vi "GL Center.vi"(5 "Simple":bool, 6 "error in":errorcluster, 8 "Axis":T1 items=["Axis 1", "Axis 2", "Axis 3", "Axis 4", "Axis 5", "Axis 6", "Axis 7", "Axis 8"], 9 "Galil.IGalil":refnum<k7>) -> (0 "error out":errorcluster, 2 "Axis Out":T1 items=["Axis 1", "Axis 2", "Axis 3", "Axis 4", "Axis 5", "Axis 6", "Axis 7", "Axis 8"], 3 "Galil Out":refnum<k7>)   [LabVIEW 2022 SP3]
doc: "Sets the operation mode for an axis or vector space."
uses:
  GL Axis Control.ctl
  Command Menu.ctl
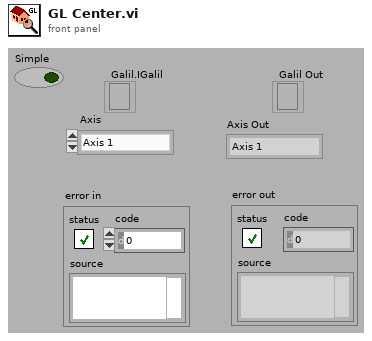
[diagram p1: front panel]
types:
  T1 = typedef "GL Axis Control.ctl" = u16
  T2 = enum16{"Absolute Position", "Relative Position", "Velocity", "Relative to Cap Pos", "Modulus Position", "Absolute Contouring", "Relative Contouring"}
  T3 = typedef "Command Menu.ctl" = enum16{"CommandPassThrough", "Abort Motion", "Define Pos", "Velocity", "Acceleration", "Deceleration", "Position Rel", "Postion Abs", "Begin Move", "After Move", "Home", "KI", "KD", "KP", "IL", "Config I/O", "Set Bit", "Clear Bit", "Motor Off", "Moto On", "Status", "Execute", "Halt Execute", "HX Status", "Tell Velocity", "Check Motion", "BreakPoint", "Tell Position", "Current Code Line", "Tell Switches", "OC Force On", "OC Off", "Pos Soft Limit", "Rev Soft Limit"}
  T4 = cluster{"HomeStatus":bool, "ReverseLimit?":bool, "ForwardLimit?":bool, "LimitHit?":bool, "MotorOff?":bool, "Motion?":bool}
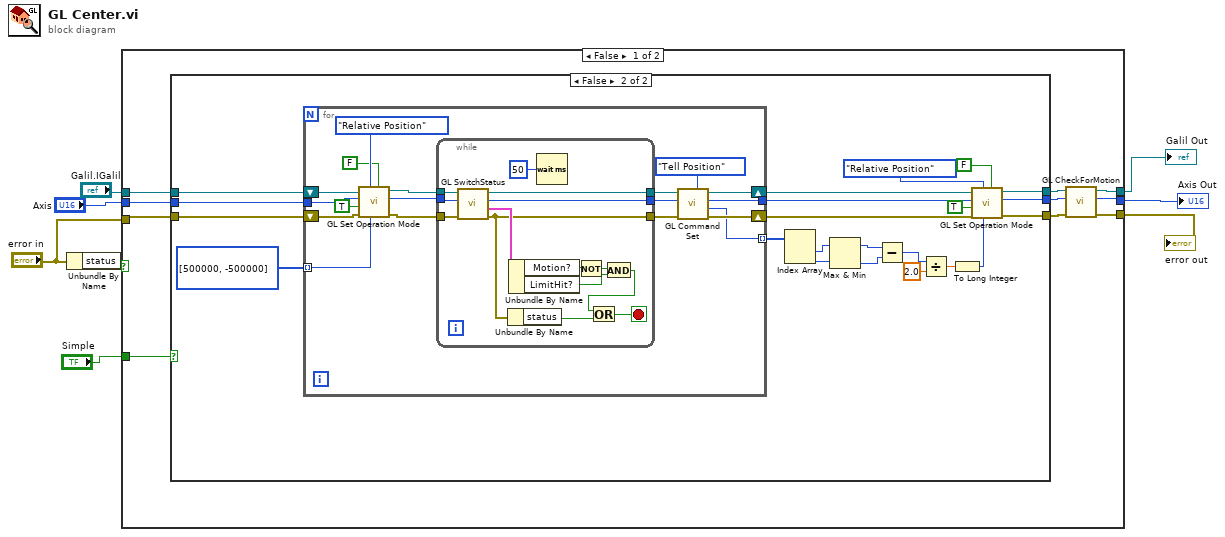
[diagram p0: block diagram]
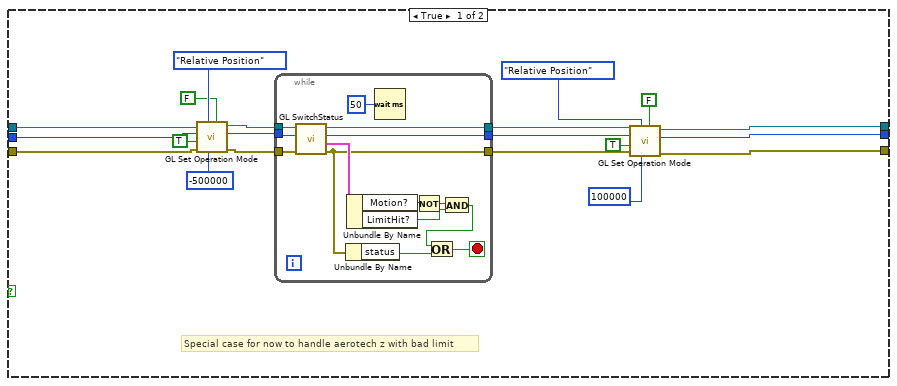
[diagram p2: hidden frame]
diagram:
  n1 = Unbundle By Name("error in") -> ("status"=w7:bool)
  n2 = case shown="False" w7 {
    tunnel: "error in" -> [w18 w109]
    tunnel: [w11 w109] -> w8
    tunnel: [w12 w108] -> w6
    tunnel: "Galil.IGalil" -> [w17 w108]
    tunnel: "Axis" -> [w16 w107]
    tunnel: [w10 w107] -> w3
    tunnel: "Simple" -> [w15 _]
    frame False {
      n3 = case shown="False" w15 {
        tunnel: w18 -> [w38 w74]
        tunnel: w17 -> [w37 w65]
        tunnel: w16 -> [w36 w64]
        tunnel: [w34 w57] -> w9
        tunnel: [w33 w56] -> w14
        tunnel: [w32 w55] -> w13
        frame True {
          # "Special case for now to handle aerotech z with bad limit"
          n4 = call "GL Set Operation Mode.vi"("LimitWarning?"=FALSE, "position cts (abs/rel)"=-500000, "Position Mode (Absolute)"=T2."Relative Position", "error in (no error)"=w38, "Start Now?"=TRUE, "Axis"=w36, "Galil.IGalil"=w37) -> ("error out"=w27:errorcluster, "Axis Out Output"=w26:T1, "Galil Out"=w28:refnum<k7>)  [unwired: 2 in]
          n5 = while {
            tunnel: w28 -> [w52]
            tunnel: [w50] -> w21
            tunnel: [w45] -> w20
            tunnel: w27 -> [w51]
            tunnel: w26 -> [w49]
            tunnel: [w48] -> w19
            stop <- w43 stop-if-true
            n6 = call "GL SwitchStatus.vi"("error in (no error)"=w51, "Axis"=w49, "Galil.IGalil"=w52) -> ("error out"=w45:errorcluster, "TS Status"=w47:T4, "Axis Out"=w48:T1, "ref out"=w50:refnum<k7>)  [unwired: 3 in]
            n7 = Unbundle By Name(w45) -> ("status"=w44:bool)
            n8 = Unbundle By Name(w47) -> ("Motion?"=w42:bool, "LimitHit?"=w40:bool)
            n9 = Wait (ms)(milliseconds to wait=u32 50) -> ()  [unwired: 1 out]
            n10 = Not(x=w42) -> (.not. x?=w41:bool)
            n11 = And(x=w41, y=w40) -> (x .and. y?=w39:bool)
            n12 = Or(x=w39, y=w44) -> (x .or. y?=w43:bool)
          }
          n13 = call "GL Set Operation Mode.vi"("LimitWarning?"=FALSE, "position cts (abs/rel)"=100000, "Position Mode (Absolute)"=T2."Relative Position", "error in (no error)"=w20, "Start Now?"=TRUE, "Axis"=w19, "Galil.IGalil"=w21) -> ("error out"=w32:errorcluster, "Axis Out Output"=w34:T1, "Galil Out"=w33:refnum<k7>)  [unwired: 2 in]
        }
        frame False {
          n14 = for {
            tunnel: [w85] -> w73 mode=indexing
            shift-right: [w90] -> w62
            shift-left: w65 -> [w80]
            shift-right: [w88] -> w61
            shift-left: w74 -> [w81]
            tunnel: w64 -> [w78]
            tunnel: [w86] -> w58
            tunnel: i32[] [500000, -500000] -> [w77] mode=indexing
            n15 = call "GL Set Operation Mode.vi"("LimitWarning?"=FALSE, "position cts (abs/rel)"=w77, "Position Mode (Absolute)"=T2."Relative Position", "error in (no error)"=w81, "Start Now?"=TRUE, "Axis"=w78, "Galil.IGalil"=w80) -> ("error out"=w82:errorcluster, "Axis Out Output"=w79:T1, "Galil Out"=w83:refnum<k7>)  [unwired: 2 in]
            n16 = while {
              tunnel: w83 -> [w106]
              tunnel: [w104] -> w91
              tunnel: [w99] -> w89
              tunnel: w82 -> [w105]
              tunnel: w79 -> [w103]
              tunnel: [w102] -> w87
              stop <- w97 stop-if-true
              n17 = call "GL SwitchStatus.vi"("error in (no error)"=w105, "Axis"=w103, "Galil.IGalil"=w106) -> ("error out"=w99:errorcluster, "TS Status"=w101:T4, "Axis Out"=w102:T1, "ref out"=w104:refnum<k7>)  [unwired: 3 in]
              n18 = Unbundle By Name(w99) -> ("status"=w98:bool)
              n19 = Unbundle By Name(w101) -> ("Motion?"=w96:bool, "LimitHit?"=w94:bool)
              n20 = Wait (ms)(milliseconds to wait=u32 50) -> ()  [unwired: 1 out]
              n21 = Not(x=w96) -> (.not. x?=w95:bool)
              n22 = And(x=w95, y=w94) -> (x .and. y?=w93:bool)
              n23 = Or(x=w93, y=w98) -> (x .or. y?=w97:bool)
            }
            n24 = call "GL Command Set.vi"("Command"=Command_Menu."Tell Position", "error in (no error)"=w89, "Axis"=w87, "Galil.IGalil"=w91) -> ("error out"=w88:errorcluster, "Response#"=w85:i32, "Axis Out"=w86:T1, "ref out"=w90:refnum<k7>)  [unwired: 3 in, 1 out]
          }
          n25 = Index Array(array=w73) -> (element #1=w72:i32, element #2=w71:i32)  [unwired: 2 in]
          n26 = Max & Min(x=w72, y=w71) -> (max(x,y)=w70:i32, min(x,y)=w69:i32)
          n27 = Subtract(x=w70, y=w69) -> (x-y=w68:i32)
          n28 = Divide(x=w68, y=2.0) -> (x/y=w66:dbl)
          n29 = To Long Integer(number=w66) -> (32bit integer=w60:i32)
          n30 = call "GL Set Operation Mode.vi"("LimitWarning?"=FALSE, "position cts (abs/rel)"=w60, "Position Mode (Absolute)"=T2."Relative Position", "error in (no error)"=w61, "Start Now?"=TRUE, "Axis"=w58, "Galil.IGalil"=w62) -> ("error out"=w55:errorcluster, "Axis Out Output"=w57:T1, "Galil Out"=w56:refnum<k7>)  [unwired: 2 in]
        }
      }
      n31 = call "GL CheckForMotion.vi"("error in"=w13, "Axis"=w9, "Refnum in"=w14) -> ("error out"=w11:errorcluster, "Axis out"=w10:T1, "Refnum out"=w12:refnum<k7>)  [unwired: 6 in]
    }
    frame True {
    }
  }
  "error out" <- w8
  "Galil Out" <- w6
  "Axis Out" <- w3
